vi "Open Network Stream.vi"(0 "video in":refnum<class "MSC Video.lvclass">, 1 "Network Address":string, 5 "error in (no error)":errorcluster) -> (14 "video out":refnum<class "MSC Video.lvclass">, 19 "error out":errorcluster)   [LabVIEW 2014, in "MSC Video.lvclass"]
doc: "Starts a video network stream from the selected address.\n\nIf your address needs authentification you can use the following syntax:\nPROTOCOL://USER:PASSWORD@IP/\nExample:\nrtsp://admin:password@192.168.0.30/\n\nDue to licensing limitations, it is neccssary to copy \"opencv_ffmpeg*.dll\" to either your application directory or systems folder if you want to use the h264 codec used by many network devices."
uses:
  MSC Video.lvclass
  MSC Video.lvclass/MSC Video.ctl
  Dependencies/x86/MSC I Process32.dll
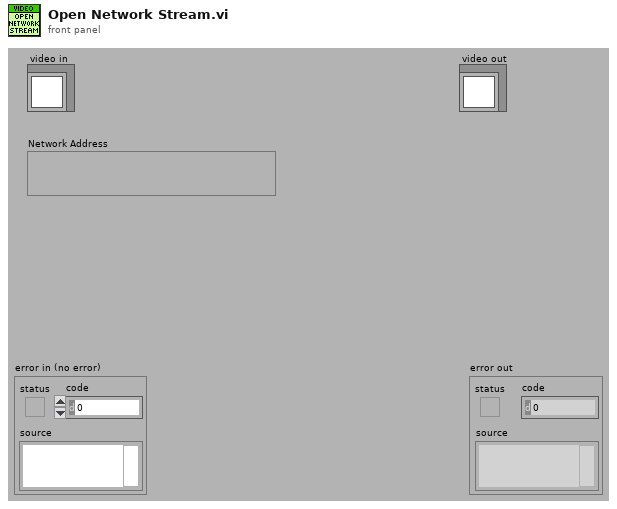
[diagram p1: front panel]
types:
  T1 = typedef "MSC Video.lvclass/Video.ctl" = cluster{"Pointer":u64, "CamID":i32, "File Path":path, "Network Address":string, "opened":bool}
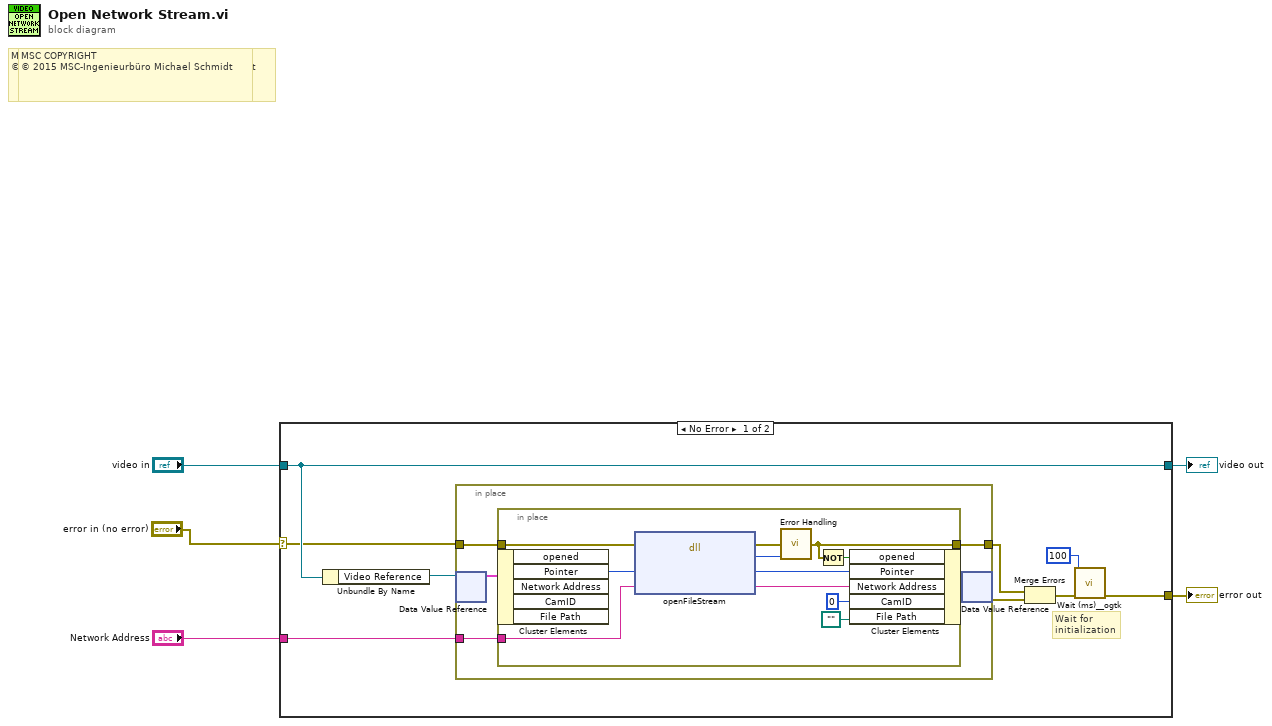
[diagram p0: block diagram]
diagram:
  # "MSC COPYRIGHT\n© 2016 MSC-Ingenieurbüro Michael Schmidt"
  # "MSC COPYRIGHT\n© 2016 MSC-Ingenieurbüro Michael Schmidt"
  # "MSC COPYRIGHT\n© 2015 MSC-Ingenieurbüro Michael Schmidt"
  n1 = case shown="No Error" "error in (no error)" {
    selector: "error in (no error)" -> [w10 w32]
    tunnel: [w9 w32] -> w4
    tunnel: "video in" -> [w11 w31]
    tunnel: [w11 w31] -> w2
    tunnel: "Network Address" -> [w6 _]
    frame No Error {
      # "Wait for\ninitialization"
      n2 = Unbundle By Name(w11) -> ("Video Reference"=w12:refnum<data-value>)
      n3 = in-place {
        in-place-border: [w17] -> w13
        in-place-border: w6 -> [w16]
        in-place-border: w10 -> [w15]
        n4 = in-place-dvr #1(w12) -> (w18:T1)  [unwired: 1 out]
        n5 = in-place {
          in-place-border: [w26] -> w17
          in-place-border: w16 -> [w29]
          in-place-border: w15 -> [w23]
          n6 = in-place-cluster #2(w18) -> ("Pointer"=w30:u64)  [unwired: 4 out]
          n7 = dll-call lib="C:/Users/MSC/LabVIEW Projekte/LV 2014/MSC I-Process/user.lib/MSC-I Process/Dependencies/x86/MSC I Process*.dll" fn="openFileStream"(error in=w23, "pointer"=w30, "fileString"=w29) -> (error out=w28:errorcluster, "error"=w27:i32, "pointer"=w24:u64, "fileString"=w21:string)  [unwired: 2 in, 1 out]
          n8 = call "Error Handling.vi"("error in (no error)"=w28, "return type"=w27) -> ("error out"=w26:errorcluster)  [unwired: 12 in, 1 out]
          n9 = Not(x=w26) -> (.not. x?=w25:bool)
          n10 = in-place-cluster #2("opened"=w25, "Pointer"=w24, "Network Address"=w21, "CamID"=0, "File Path"=path "") -> (w19:T1)
        }
        n11 = in-place-dvr #1(w19) -> (w14:errorcluster)  [unwired: 1 out]
      }
      n12 = Merge Errors(w13, w14) -> (w8:errorcluster)
      n13 = call <userlib>:"Wait (ms)__ogtk.vi"("error in (no error)"=w8, "milliseconds to wait"=u32 100) -> ("error out"=w9:errorcluster)  [unwired: 8 in, 1 out]
    }
    frame Error {
    }
  }
  "error out" <- w4
  "video out" <- w2
